vi "Get Parent State.vi"(8 "error in (no error)":errorcluster, 10 "Boolean":bool, 11 "Child Actor in":refnum<class "Child Actor.lvclass">) -> (0 "error out":errorcluster, 3 "Child Actor out":refnum<class "Child Actor.lvclass">)   [LabVIEW 2012, in "Child Actor.lvclass"]
uses:
  Child Actor.lvclass
  Child Actor.lvclass/Child Actor.ctl
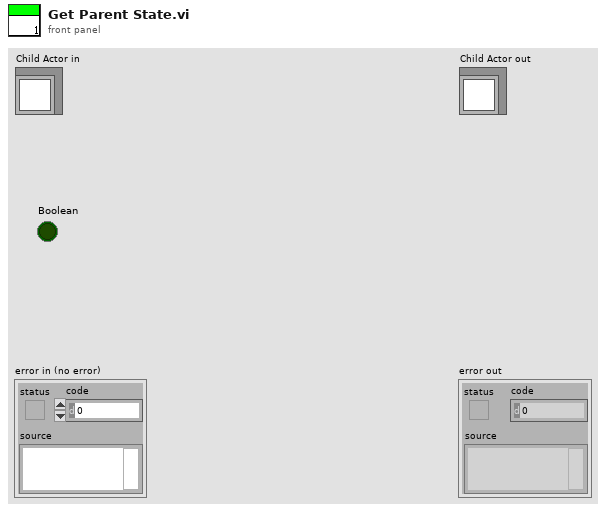
[diagram p1: front panel]
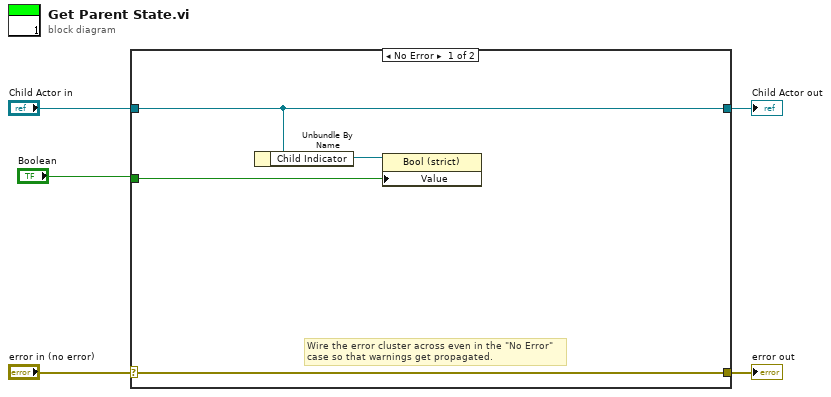
[diagram p0: block diagram]
diagram:
  n1 = case shown="No Error" "error in (no error)" {
    selector: "error in (no error)" -> [w9 w11]
    tunnel: [w9 w11] -> w4
    tunnel: [w8 w10] -> w2
    tunnel: "Child Actor in" -> [w8 w10]
    tunnel: "Boolean" -> [w6 _]
    frame No Error {
      # "Wire the error cluster across even in the \"No Error\"\ncase so that warnings get propagated."
      n2 = Unbundle By Name(w8) -> ("Child Indicator"=w7:refnum<vi>)
      n3 = property class="Bool (strict)"(reference=w7, "Value"=w6) -> ()  [unwired: 1 in, 2 out]
    }
    frame Error {
    }
  }
  "error out" <- w4
  "Child Actor out" <- w2
